vi "Get Outline Box.vi"(7 "BBox (True)":bool=TRUE, 8 "error in (no error)":errorcluster, 11 "contour glyph ref":i64) -> (0 "error out":errorcluster, 1 "Size":cluster{"width":sgl, "height":sgl}, 2 "Box":T1, 3 "contour glyph ref dup":i64)   [LabVIEW 2023, in "Freetype Drawer.lvlib"]
uses:
  Freetype Drawer.lvlib
  libfreetype.dll
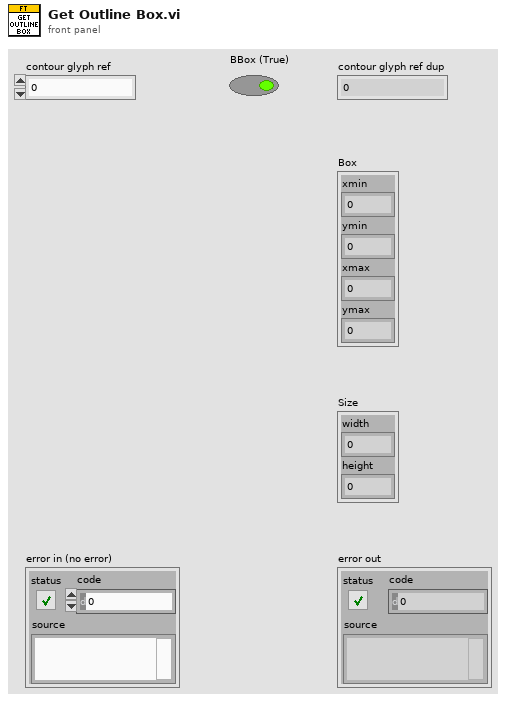
[diagram p1: front panel]
types:
  T1 = cluster{"xmin":sgl, "ymin":sgl, "xmax":sgl, "ymax":sgl}
  T2 = cluster{"xmin":i32, "ymin":i32, "xmax":i32, "ymax":i32}
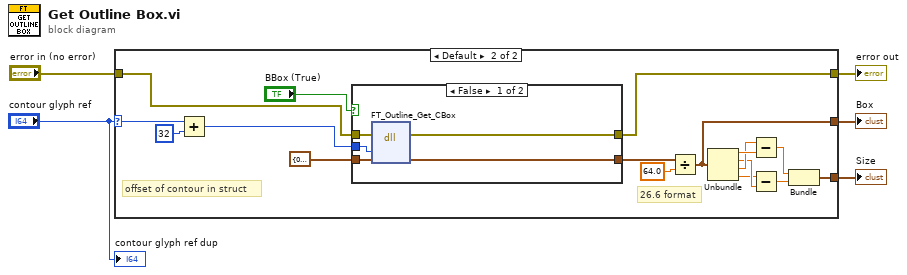
[diagram p0: block diagram]
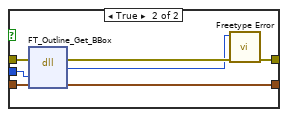
[diagram p3: hidden frame]
diagram:
  n1 = case shown="Default" "contour glyph ref" {
    selector: "contour glyph ref" -> [_ w10]
    tunnel: "error in (no error)" -> [w6 w11]
    tunnel: [w6 w23] -> w4
    tunnel: [_ w20] -> w3
    tunnel: [_ w13] -> w2
    frame 0 {
    }
    frame Default {
      # "26.6 format"
      # "offset of contour in struct"
      n2 = Add(x=w10, y=i64 32) -> (x+y=w9:i64)
      n3 = case shown="False" "BBox (True)" {
        tunnel: T2 {"xmin"=0, "ymin"=0, "xmax"=0, "ymax"=0} ("bbox") -> [w26 w35]
        tunnel: [w25 w34] -> w21
        tunnel: w11 -> [w28 w33]
        tunnel: [w27 w31] -> w23
        tunnel: w9 -> [w24 w29]
        frame False {
          n4 = dll-call lib="E:/Labview/LV 2023/Libs/LV Symbol/Freetype Drawer/Wrappers/libfreetype.dll" fn="FT_Outline_Get_CBox"(error in=w28, "outline"=w24, "box"=w26) -> (error out=w27:errorcluster, "box"=w25:T2)  [unwired: 4 in, 1 out]
        }
        frame True {
          n5 = dll-call lib="E:/Labview/LV 2023/Libs/LV Symbol/Freetype Drawer/Wrappers/libfreetype.dll" fn="FT_Outline_Get_BBox"(error in=w33, "outline"=w29, "box"=w35) -> (error out=w32:errorcluster, "return type"=w30:i32, "box"=w34:T2)  [unwired: 3 in, 1 out]
          n6 = call "Freetype Error.vi"("error in (no error)"=w32, "Error"=w30) -> ("error out"=w31:errorcluster)  [unwired: 9 in]
        }
      }
      n7 = Divide(x=w21, y=sgl 64.0) -> (x/y=w20:T1)
      n8 = Unbundle(w20) -> ("xmin"=w19:sgl, "ymin"=w17:sgl, "xmax"=w18:sgl, "ymax"=w16:sgl)
      n9 = Subtract(x=w18, y=w19) -> (x-y=w14:sgl)
      n10 = Subtract(x=w16, y=w17) -> (x-y=w15:sgl)
      n11 = Bundle(w14, w15) -> (w13:cluster{sgl, sgl})  [unwired: 1 in]
    }
  }
  "Box" <- w3
  "error out" <- w4
  "Size" <- w2
  "contour glyph ref dup" <- "contour glyph ref"
